vi "SERIAL_GetSetRefnum.vi"(8 "error in (no error)":errorcluster, 9 "menu":enum16{"set", "get", "delete"}(ring), 10 "refnum name":string, 11 "navX DevRef":T1={"SerialPortRef"={"DevStatus"={"status"=FALSE, "code"=0, "source"=""}, "Serial Port Name"=""}, "Board Information"={"WhoAmI (50 | 0x32)"=0, "Board Revision"=0, "Firmware Major Version"=0, "Firmware Minor Version"=0, "NAVX_BOARD_CAPABILITY"={"OMNIMOUNT"=FALSE, "YAW_RESET"=FALSE, "VEL_AND_DISP"=FALSE}, "NAVX_BOARD_YAW_AXIS"={"BOARD_YAW_AXIS_UP"=FALSE, "BOARD_YAW_AXIS"=0}}, "Status"={"Update Rate Hz"=0, "Accelerometer Full-Scale Range"=0, "Gyro Full-Scale Range"=0, "NAVX_OP_STATUS"=0, "NAVX_CAL_STATUS"=0, "NAVX_SELFTEST_STATUS"=0, "NAVX_SENSOR_STATUS"={"MOVING"=FALSE, "YAW_STABLE"=FALSE, "MAG_DISTURBANCE"=FALSE, "ALTITUDE_VALID"=FALSE, "SEALEVEL_PRESS_SET"=FALSE, "FUSED_HEADING_VALID"=FALSE}}, "Offsets"={"Yaw"=0.0, "Quat W"=0.0, "Quat X"=0.0, "Quat Y"=0.0, "Quat Z"=0.0}, "Update Rate (4Hz-60Hz)"=50, "Nav6Mode (YPR)"=enum."YPR", "refnum name"="", "error"={"status"=FALSE, "code"=0, "source"=""}, "Loop VI Refnum"=refnum} {"Status"."NAVX_OP_STATUS" items=["INITIALIZING", "SELFTEST_IN_PROGRESS", "ERROR", "IMU_AUTOCAL_IN_PROGRESS", "NORMAL"]; "Status"."NAVX_CAL_STATUS" items=["IMU_CAL_STATE_MASK"=3, "IMU_CAL_INPROGRESS"=0, "IMU_CAL_ACCUMULATE"=1, "IMU_CAL_COMPLETE"=2, "MAG_CAL_COMPLETE"=4, "BARO_CAL_COMPLETE"=8]}) -> (0 "error out":errorcluster, 3 "navX DevRef":T1={"SerialPortRef"={"DevStatus"={"status"=FALSE, "code"=0, "source"=""}, "Serial Port Name"=""}, "Board Information"={"WhoAmI (50 | 0x32)"=0, "Board Revision"=0, "Firmware Major Version"=0, "Firmware Minor Version"=0, "NAVX_BOARD_CAPABILITY"={"OMNIMOUNT"=FALSE, "YAW_RESET"=FALSE, "VEL_AND_DISP"=FALSE}, "NAVX_BOARD_YAW_AXIS"={"BOARD_YAW_AXIS_UP"=FALSE, "BOARD_YAW_AXIS"=0}}, "Status"={"Update Rate Hz"=0, "Accelerometer Full-Scale Range"=0, "Gyro Full-Scale Range"=0, "NAVX_OP_STATUS"=0, "NAVX_CAL_STATUS"=0, "NAVX_SELFTEST_STATUS"=0, "NAVX_SENSOR_STATUS"={"MOVING"=FALSE, "YAW_STABLE"=FALSE, "MAG_DISTURBANCE"=FALSE, "ALTITUDE_VALID"=FALSE, "SEALEVEL_PRESS_SET"=FALSE, "FUSED_HEADING_VALID"=FALSE}}, "Offsets"={"Yaw"=0.0, "Quat W"=0.0, "Quat X"=0.0, "Quat Y"=0.0, "Quat Z"=0.0}, "Update Rate (4Hz-60Hz)"=50, "Nav6Mode (YPR)"=enum."YPR", "refnum name"="", "error"={"status"=FALSE, "code"=0, "source"=""}, "Loop VI Refnum"=refnum} {"Status"."NAVX_OP_STATUS" items=["INITIALIZING", "SELFTEST_IN_PROGRESS", "ERROR", "IMU_AUTOCAL_IN_PROGRESS", "NORMAL"]; "Status"."NAVX_CAL_STATUS" items=["IMU_CAL_STATE_MASK"=3, "IMU_CAL_INPROGRESS"=0, "IMU_CAL_ACCUMULATE"=1, "IMU_CAL_COMPLETE"=2, "MAG_CAL_COMPLETE"=4, "BARO_CAL_COMPLETE"=8]})   [LabVIEW 2014, in "navX-MXP IMU.lvlib"]
uses:
  navX-MXP IMU.lvlib
  Internal/navX Serial DevRef.ctl
  <vilib>/Rock Robotics/WPI/SerialPort/WPI_SerialPortRef.ctl
  COMMON/TypeDefs/Data TypeDefs/navX Board Information.ctl
  COMMON/TypeDefs/Value TypeDefs/navX NAVX_BOARD_CAPABILITY.ctl
  COMMON/TypeDefs/Value TypeDefs/navX NAVX_BOARD_YAW_AXIS.ctl
  COMMON/TypeDefs/Data TypeDefs/navX Status Data.ctl
  COMMON/TypeDefs/Value TypeDefs/navX NAVX_OP_STATUS.ctl
  COMMON/TypeDefs/Value TypeDefs/navX NAVX_CAL_STATUS.ctl
  COMMON/TypeDefs/Value TypeDefs/navX NAVX_SENSOR_STATUS.ctl
  TypeDefs/navX Serial Mode.ctl
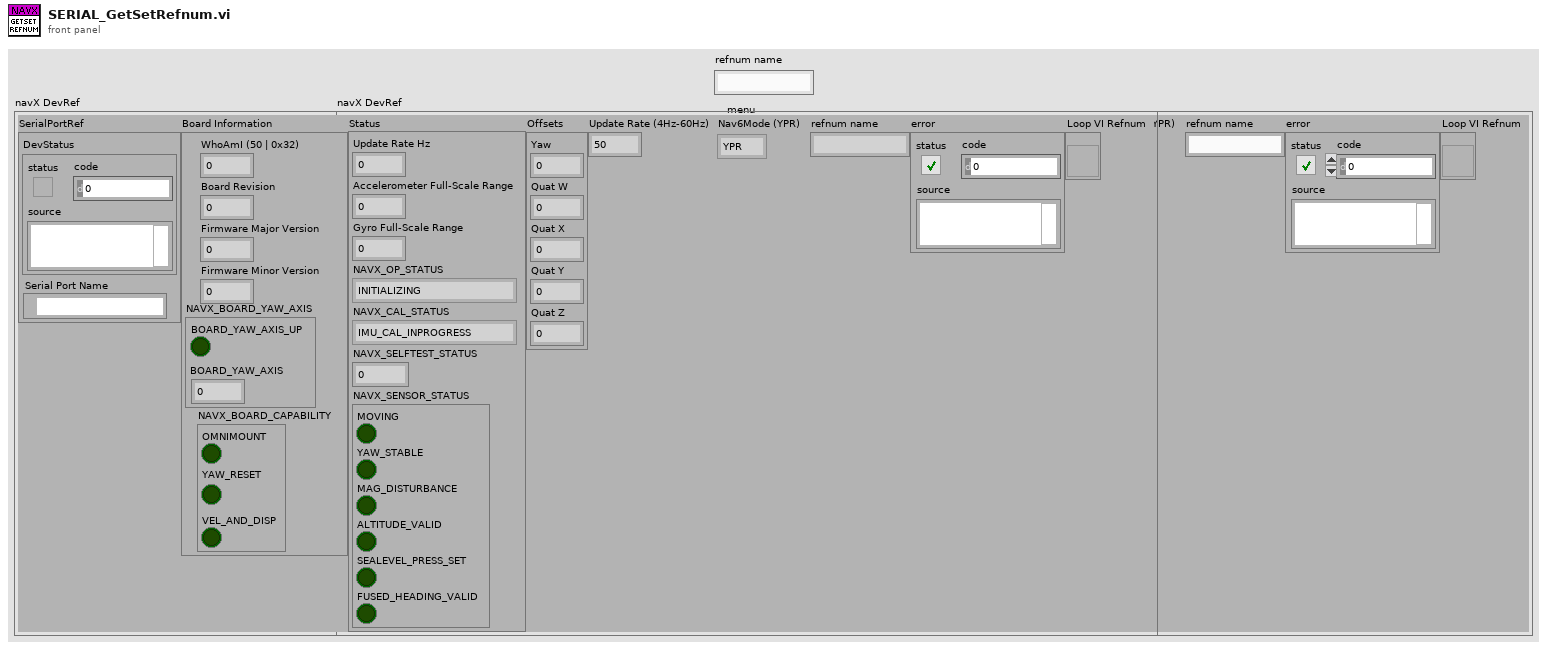
[diagram p1: front panel]
types:
  T1 = typedef "navX-MXP IMU.lvlib/navX Serial DevRef.ctl" = cluster{"SerialPortRef":T2, "Board Information":T3, "Status":T6, "Offsets":cluster{"Yaw":dbl, "Quat W":dbl, "Quat X":dbl, "Quat Y":dbl, "Quat Z":dbl}, "Update Rate (4Hz-60Hz)":u8, "Nav6Mode (YPR)":T10, "refnum name":string, "error":errorcluster, "Loop VI Refnum":refnum<vi>}
  T2 = typedef "WPI_SerialPortRef.ctl" = cluster{"DevStatus":errorcluster, "Serial Port Name":refnum<visa-resource-name>}
  T3 = typedef "navX-MXP IMU.lvlib/navX Board Information.ctl" = cluster{"WhoAmI (50 | 0x32)":u8, "Board Revision":u8, "Firmware Major Version":u8, "Firmware Minor Version":u8, "NAVX_BOARD_CAPABILITY":T4, "NAVX_BOARD_YAW_AXIS":T5}
  T4 = typedef "navX-MXP IMU.lvlib/navX NAVX_BOARD_CAPABILITY.ctl" = cluster{"OMNIMOUNT":bool, "YAW_RESET":bool, "VEL_AND_DISP":bool}
  T5 = typedef "navX-MXP IMU.lvlib/navX NAVX_BOARD_YAW_AXIS.ctl" = cluster{"BOARD_YAW_AXIS_UP":bool, "BOARD_YAW_AXIS":u8}
  T6 = typedef "navX-MXP IMU.lvlib/navX Status Data.ctl" = cluster{"Update Rate Hz":u8, "Accelerometer Full-Scale Range":u8, "Gyro Full-Scale Range":u16, "NAVX_OP_STATUS":T7, "NAVX_CAL_STATUS":T8, "NAVX_SELFTEST_STATUS":u8, "NAVX_SENSOR_STATUS":T9}
  T7 = typedef "navX-MXP IMU.lvlib/navX NAVX_OP_STATUS.ctl" = u8
  T8 = typedef "navX-MXP IMU.lvlib/navX NAVX_CAL_STATUS.ctl" = u8
  T9 = typedef "navX-MXP IMU.lvlib/navX NAVX_SENSOR_STATUS.ctl" = cluster{"MOVING":bool, "YAW_STABLE":bool, "MAG_DISTURBANCE":bool, "ALTITUDE_VALID":bool, "SEALEVEL_PRESS_SET":bool, "FUSED_HEADING_VALID":bool}
  T10 = typedef "navX-MXP IMU.lvlib/navX Serial Mode.ctl" = enum16{"YPR", "Gyro", "Quaternion"}
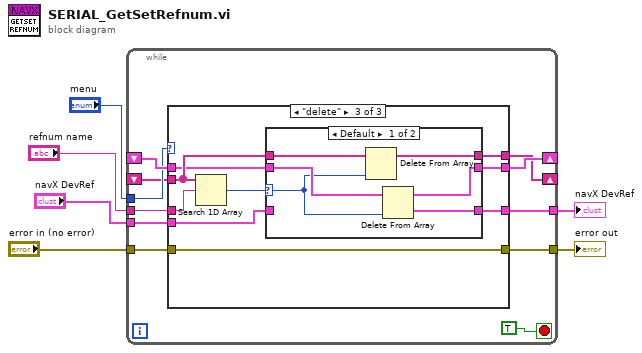
[diagram p0: block diagram]
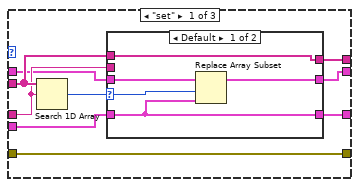
[diagram p2: hidden frame]
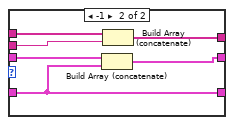
[diagram p3: hidden frame]
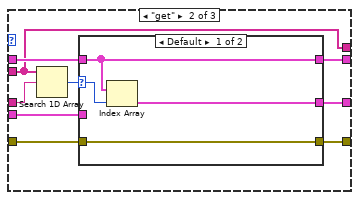
[diagram p4: hidden frame]
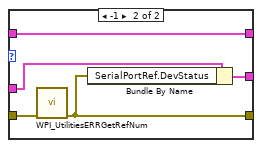
[diagram p5: hidden frame]
diagram:
  n1 = while {
    tunnel: "navX DevRef" -> [w17]
    tunnel: "refnum name" -> [w10]
    tunnel: "error in (no error)" -> [w9]
    shift-right: [w16] -> _
    shift-left: _ -> [w15]
    tunnel: [w14] -> w1
    tunnel: "menu" -> [w13]
    shift-right: [w12] -> _
    shift-left: _ -> [w11]
    tunnel: [w8] -> w4
    stop <- TRUE stop-if-true
    n2 = case shown="\"delete\"" w13 {
      tunnel: w17 -> [w21 w43 w59]
      tunnel: [w20 w42 w58] -> w16
      tunnel: w15 -> [w22 w44 w60]
      tunnel: [w19 w41 w57] -> w14
      tunnel: [w26 w40 w64] -> w12
      tunnel: w11 -> [w25 w40 w63]
      tunnel: w10 -> [w23 w45 w61]
      tunnel: [w18 w38 w56] -> w8
      tunnel: w9 -> [w18 w39 w56]
      frame "set" {
        n3 = Search 1D Array(1D array=w25, element=w23) -> (index of element=w24:i32)  [unwired: 1 out]
        n4 = case shown="Default" w24 {
          selector: w24 -> [w29 _]
          tunnel: [w31 w37] -> w26
          tunnel: w25 -> [w31 w36]
          tunnel: w23 -> [_ w35]
          tunnel: w22 -> [w30 w34]
          tunnel: w21 -> [w27 w32]
          tunnel: [w28 w33] -> w20
          tunnel: [w27 w32] -> w19
          frame Default {
            n5 = Replace Array Subset(array=w30, new element=w27, index=w29) -> (w28:T1[])
          }
          frame -1 {
            n6 = Build Array (concatenate)(w34, w32) -> (w33:T1[])
            n7 = Build Array (concatenate)(w36, w35) -> (w37:string[])
          }
        }
      }
      frame "get" {
        n8 = Search 1D Array(1D array=w40, element=w45) -> (index of element=w46:i32)  [unwired: 1 out]
        n9 = case shown="Default" w46 {
          selector: w46 -> [w50 _]
          tunnel: w44 -> [w48 w55]
          tunnel: w43 -> [_ w53]
          tunnel: [w48 w55] -> w42
          tunnel: [w49 w52] -> w41
          tunnel: w39 -> [w47 w54]
          tunnel: [w47 w51] -> w38
          frame Default {
            n10 = Index Array(array=w48, index=w50) -> (element=w49:T1)
          }
          frame -1 {
            n11 = call <vilib>:"WPI_UtilitiesERRGetRefNum.vi"("error in (no error)"=w54) -> ("ERRGetRefNum"=w51:errorcluster)  [unwired: 10 out]
            n12 = Bundle By Name(cluster=w53, "SerialPortRef.DevStatus"=w51) -> (w52:T1)
          }
        }
      }
      frame "delete" {
        n13 = Search 1D Array(1D array=w63, element=w61) -> (index of element=w62:i32)  [unwired: 1 out]
        n14 = case shown="Default" w62 {
          selector: w62 -> [w65 _]
          tunnel: [w66 w72] -> w64
          tunnel: w63 -> [w67 w72]
          tunnel: w60 -> [w70 w71]
          tunnel: w59 -> [_ w73]
          tunnel: [w69 w71] -> w58
          tunnel: [w68 w73] -> w57
          frame Default {
            n15 = Delete From Array(array=w67, index=w65) -> (array with subset deleted=w66:string[])  [unwired: 1 in, 1 out]
            n16 = Delete From Array(array=w70, index=w65) -> (deleted portion=w68:T1, array with subset deleted=w69:T1[])  [unwired: 1 in]
          }
          frame -1 {
          }
        }
      }
    }
  }
  "error out" <- w4
  "navX DevRef" <- w1
